vi "LeerArchivo.vi"(2 "error in (no error)":errorcluster, 3 "dup path":path, 4 "Conections in":T1) -> (0 "error out":errorcluster, 1 "Conections out":T1)   [LabVIEW 2016]
uses:
  <vilib>/Utility/config.llb/Read Key (String).vi
  <vilib>/Utility/config.llb/NI_LVConfig.lvlib
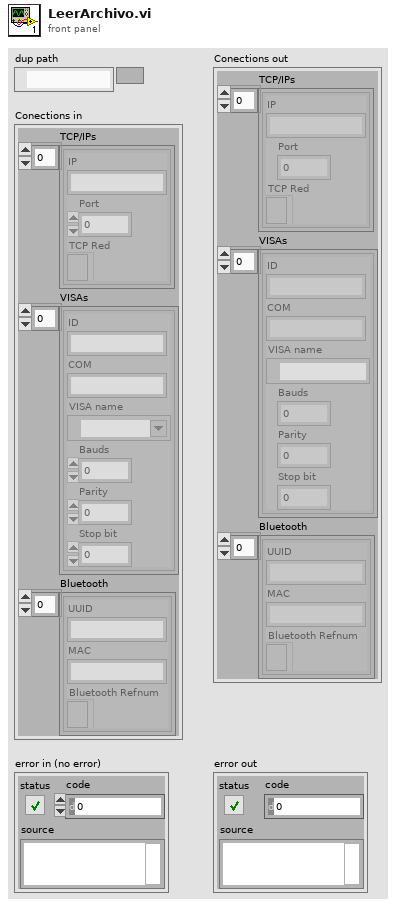
[diagram p1: front panel]
types:
  T1 = cluster{"TCP/IPs":cluster{"IP":string, "Port":u16, "TCP Red":refnum<k5>}[], "VISAs":cluster{"ID":string, "COM":string, "VISA name":refnum<visa-resource-name>, "Bauds":dbl, "Parity":u16, "Stop bit":u16}[], "Bluetooth":cluster{"UUID":string, "MAC":string, "Bluetooth Refnum":refnum<k31>}[]}
  T2 = typedef "NI_LVConfig.lvlib/Config Data RefNum.ctl" = refnum<k1>
  T3 = cluster{"ID":string, "COM":string, "VISA name":refnum<visa-resource-name>, "Bauds":dbl, "Parity":u16, "Stop bit":u16}[]
  T4 = cluster{"ID":string, "COM":string, "VISA name":refnum<visa-resource-name>, "Bauds":dbl, "Parity":u16, "Stop bit":u16}
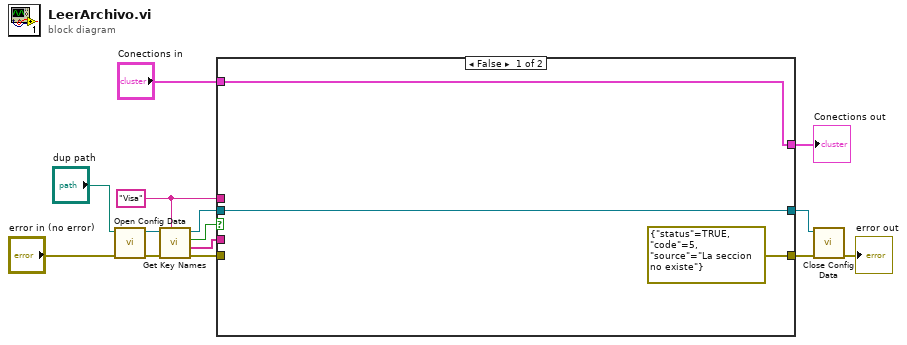
[diagram p0: block diagram]
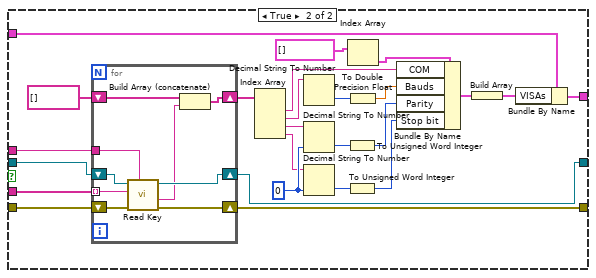
[diagram p2: hidden frame]
diagram:
  w11 = "Visa" ("section")
  n1 = call <vilib>:"Open Config Data.vi"("error in (no error)"="error in (no error)", "configuration file path"="dup path") -> ("error out"=w7:errorcluster, "refnum"=w6:T2)  [unwired: 7 in, 1 out]
  n2 = call <vilib>:"Get Key Names.vi"("section"=w11, "error in (no error)"=w7, "refnum"=w6) -> ("error out"=w9:errorcluster, "key names"=w12:string[], "section exists?"=w8:bool, "refnum out"=w10:T2)  [unwired: 5 in]
  n3 = case shown="False" w8 {
    tunnel: [errorcluster {"status"=TRUE, "code"=5, "source"="La seccion no existe"} ("error out") w34] -> w1
    tunnel: [w17 w42] -> w3
    tunnel: "Conections in" -> [w16 w41]
    tunnel: [w16 w40] -> w5
    tunnel: w9 -> [_ w39]
    tunnel: w10 -> [w17 w38]
    tunnel: w11 -> [_ w37]
    tunnel: w12 -> [_ w36]
    frame False {
    }
    frame True {
      w29 = 0
      n4 = for {
        shift-right: [w49] -> w34
        shift-left: w39 -> [w51]
        shift-right: [w48] -> w42
        shift-left: w38 -> [w50]
        tunnel: w37 -> [w47]
        tunnel: w36 -> [w46] mode=indexing
        shift-right: [w44] -> w19
        shift-left: string[] [] -> [w45]
        n5 = call-poly <vilib>:"Read Key.vi"("section"=w47, "error in (no error)"=w51, "key"=w46, "refnum"=w50) -> ("error out"=w49:errorcluster, "value"=w43:string, "refnum out"=w48:T2)  [unwired: 4 in, 1 out]
        n6 = Build Array (concatenate)(w45, w43) -> (w44:string[])
      }
      n7 = Index Array(array=w19) -> (element #1=w26:string, element #2=w23:string, element #3=w24:string, element #4=w25:string)  [unwired: 4 in]
      n8 = Decimal String To Number(string=w23) -> (number=w27:i32)  [unwired: 2 in, 1 out]
      n9 = Decimal String To Number(string=w24, default (0L)=w29) -> (number=w30:i32)  [unwired: 1 in, 1 out]
      n10 = Decimal String To Number(string=w25, default (0L)=w29) -> (number=w32:i32)  [unwired: 1 in, 1 out]
      n11 = To Unsigned Word Integer(number=w30) -> (unsigned 16bit integer=w31:u16)
      n12 = To Unsigned Word Integer(number=w32) -> (unsigned 16bit integer=w33:u16)
      n13 = Index Array(array=T3 [] ("VISAs")) -> (element=w21:T4)  [unwired: 1 in]
      n14 = To Double Precision Float(number=w27) -> (double precision float=w28:dbl)
      n15 = Bundle By Name(cluster=w21, "COM"=w26, "Bauds"=w28, "Parity"=w31, "Stop bit"=w33) -> (w20:T4)
      n16 = Build Array(w20) -> (w18:T3)
      n17 = Bundle By Name(cluster=w41, "VISAs"=w18) -> (w40:T1)
    }
  }
  "Conections out" <- w5
  n18 = call <vilib>:"Close Config Data.vi"("error in (no error)"=w1, "refnum"=w3) -> ("error out"=→"error out":errorcluster)  [unwired: 8 in, 1 out]
